vi "Original GenerateTestAllTask.vi"() -> (3 "Task Out":refnum<k21>)   [LabVIEW 2013]
uses:
  <vilib>/DAQmx/create/channels.llb/DAQmx Create Channel (AI-Voltage-Basic).vi
  <vilib>/DAQmx/create/channels.llb/DAQmx Create Channel (AI-Strain-Strain Gage).vi
  <vilib>/DAQmx/create/channels.llb/DAQmx Create Channel (AI-Position-LVDT).vi
  <vilib>/DAQmx/create/channels.llb/DAQmx Create Channel (AI-Position-RVDT).vi
  Instance           1 27Saved   GenerateTestAllTask .vi
  <resource>/objmgr/daqmx.rc
  Popups/Progress Bar Actions.ctl
panel:
  in  "Channel Path List":string[](array[string])
  out "error out":errorcluster
  in  "error in (no error)":errorcluster
  out "Name":string
  out "AI.MeasType":i32(ring)=10300 items=["Voltage"=10322, "Current"=10134, "More:Voltage:Custom with Excitation"=10323, "Frequency"=10181, "Resistance"=10278, "Temperature:Thermocouple"=10303, "Temperature:Thermistor"=10302, "Temperature:RTD"=10301, "Temperature:Built-in Sensor"=10311, "Strain Gage"=10300, "Position:LVDT"=10352, "Position:RVDT"=10353, "Accelerometer"=10356, "Sound Pressure:Microphone"=10354, "TEDS Sensor"=12531]
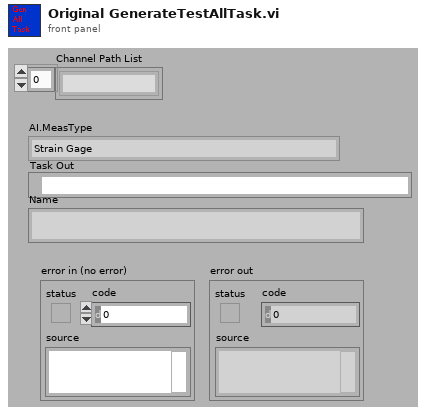
[diagram p1: front panel]
types:
  T1 = typedef "Progress Bar Actions.ctl" = enum16{"Get", "Set", "Exit", "Init"}
  T2 = cluster{"gage factor":dbl, "nominal gage resistance":dbl, "poisson ratio":dbl}
  T3 = cluster{"strain configuration":i32, "lead wire resistance":dbl, "initial bridge voltage":dbl, "voltage excitation source":i32, "voltage excitation value":dbl}
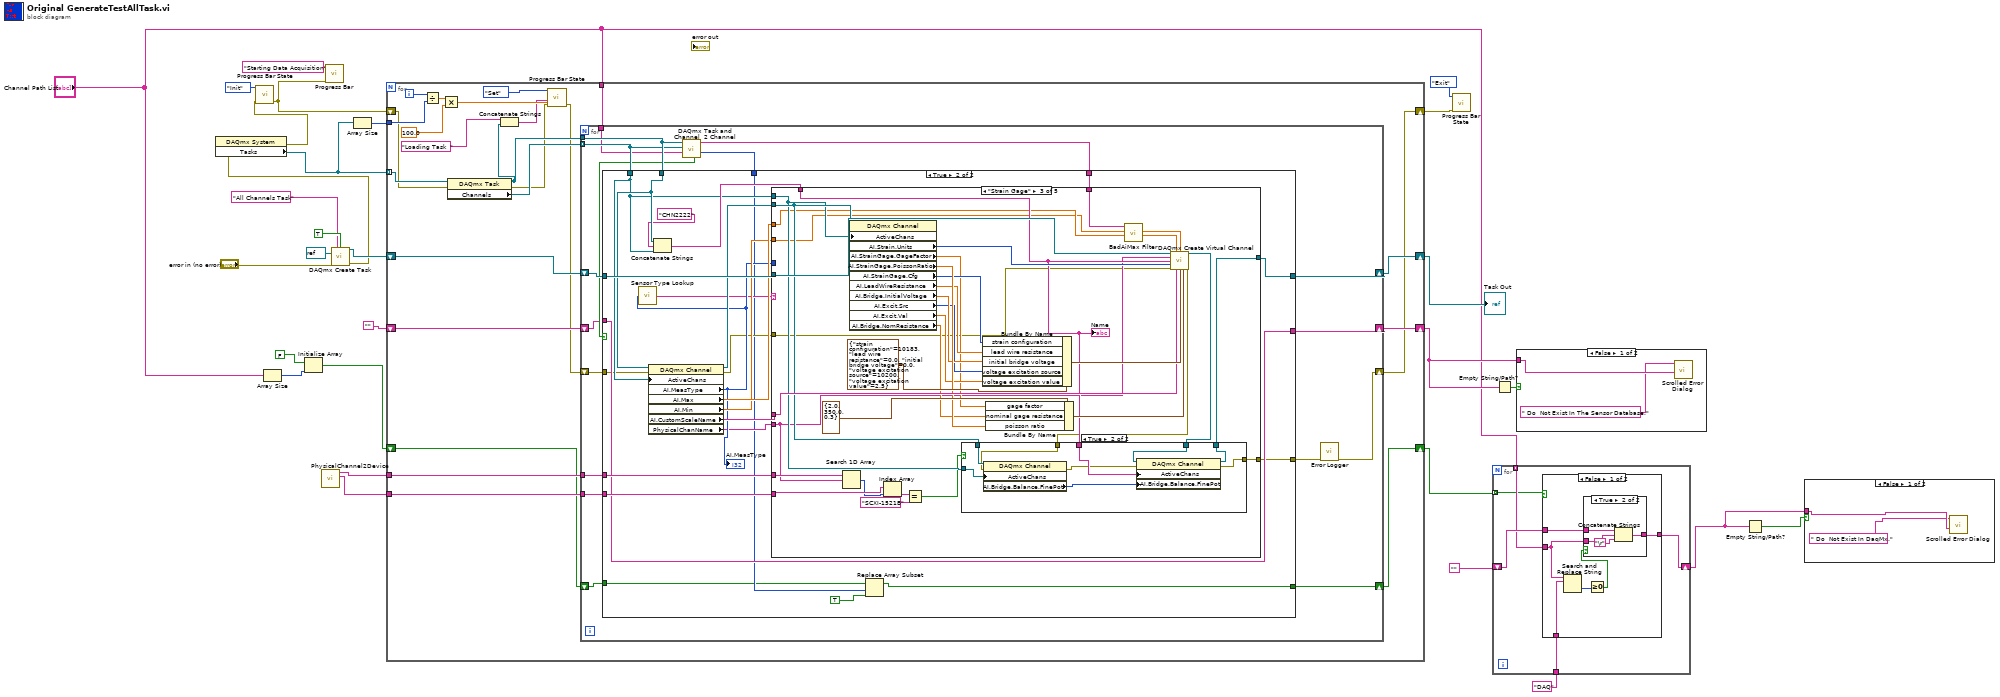
[diagram p0: block diagram]
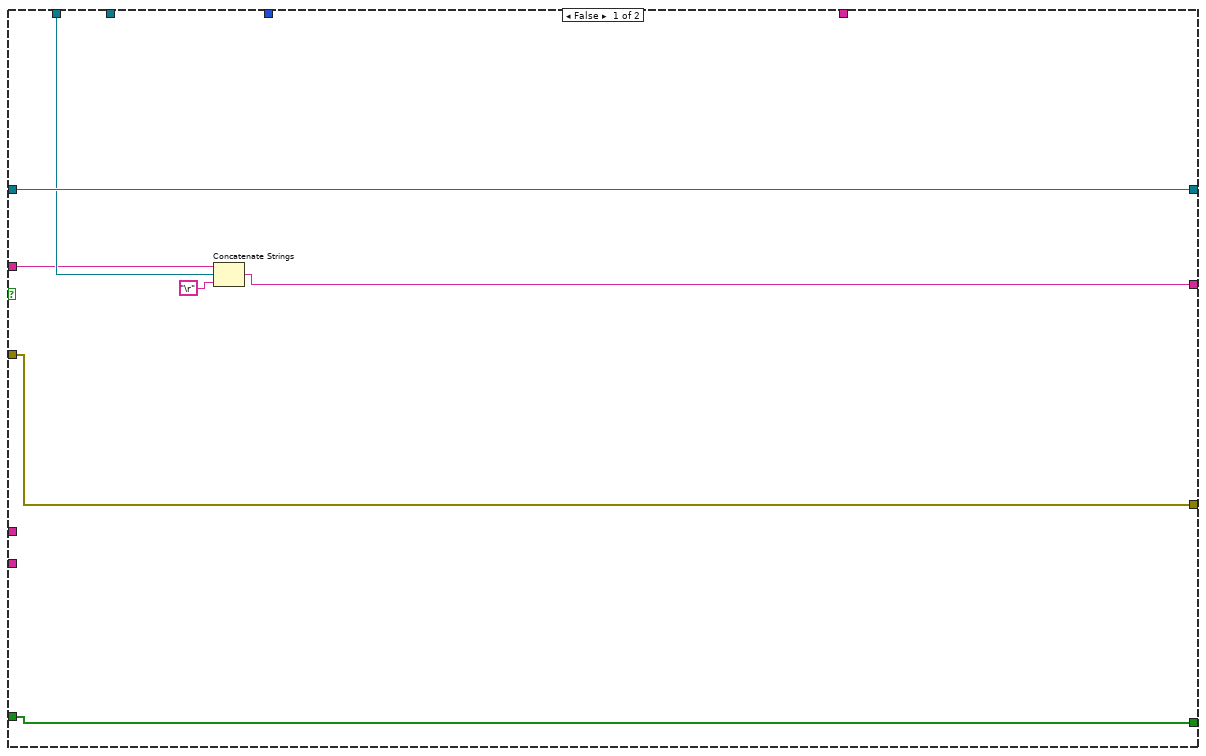
[diagram p6: hidden frame]
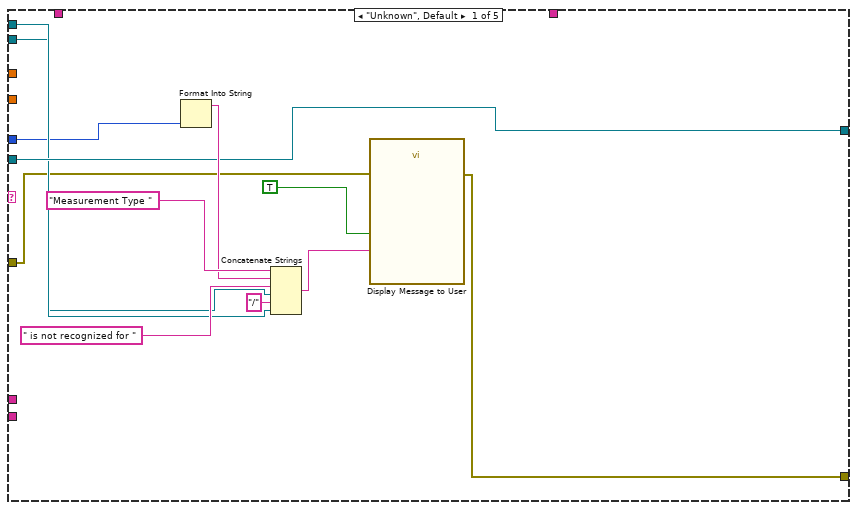
[diagram p7: hidden frame]
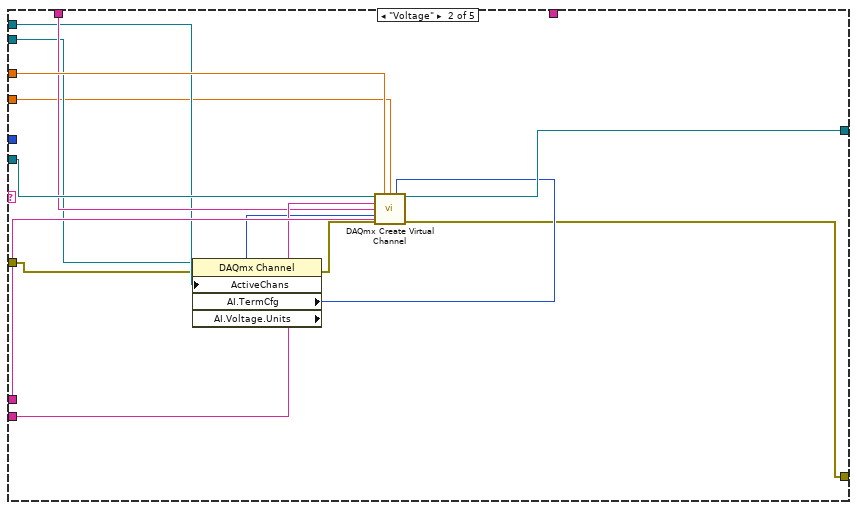
[diagram p8: hidden frame]
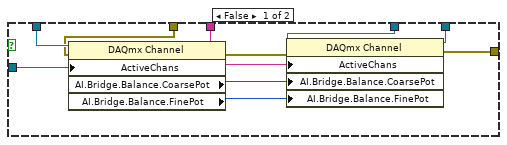
[diagram p9: hidden frame]
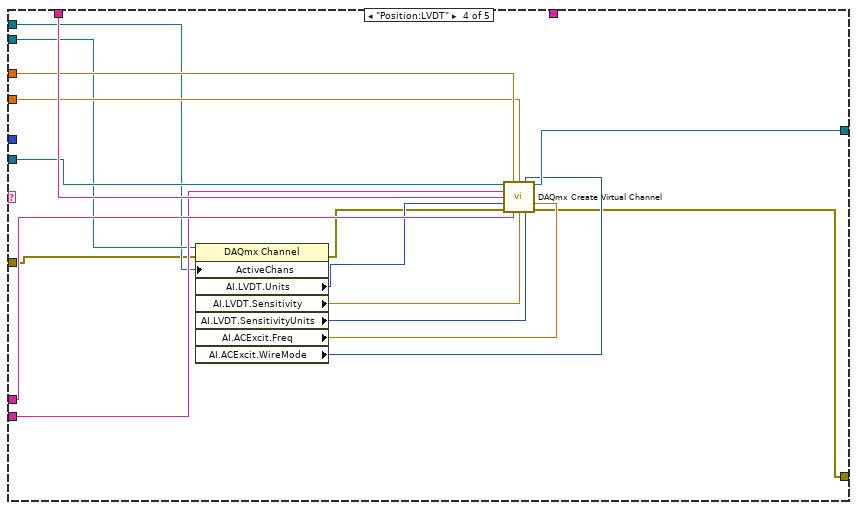
[diagram p10: hidden frame]
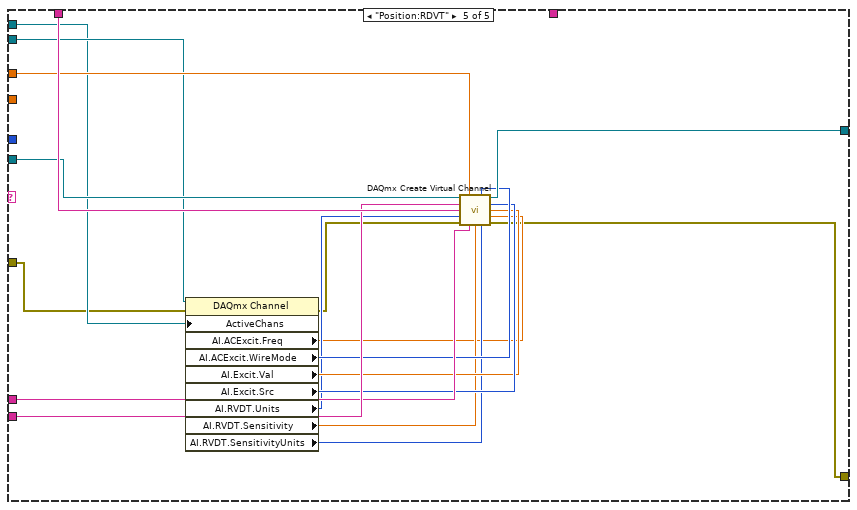
[diagram p11: hidden frame]
diagram:
  n1 = Array Size(array="Channel Path List") -> (size(s)=w10:i32)
  n2 = Initialize Array(FALSE, w10) -> (w8:bool[])
  n3 = call "PhysicalChannel2Device.vi"() -> ("Associated Device"=w23:string[], "Physical Channels"=w24:tag[])  [unwired: 10 out]
  n4 = call <vilib>:"DAQmx Create Task.vi"("new task name"="All Channels Task", "auto cleanup"=TRUE, "task to copy"=refnum<k21> refnum, "error in"="error in (no error)") -> ("task out"=w27:refnum<k21>, "error out"=w12:errorcluster)  [unwired: 1 in, 9 out]
  n5 = property class="DAQmx System"(error in=w12) -> (error out=w11:errorcluster, "Tasks"=w18:refnum<k21>[])  [unwired: 1 in, 1 out]
  n6 = call "Progress Bar State.vi"("error in (no error)"=w11, "Progress Actions"=Progress_Bar_Actions."Init") -> ("error out"=w14:errorcluster)  [unwired: 2 in, 7 out]
  n7 = call "Progress Bar.vi"("error in (no error)"=w14, "Label In"="Starting Data Acquisition") -> ()  [unwired: 10 out]
  n8 = Array Size(array=w18) -> (size(s)=w17:i32)
  n9 = for {
    tunnel: w18 -> [w53] mode=indexing
    shift-right: [w50] -> w26
    shift-left: w27 -> [w51]
    tunnel: w24 -> [w49]
    tunnel: w23 -> [w48]
    shift-right: [w46] -> w21
    shift-left: "" -> [w47]
    tunnel: w17 -> [w43]
    shift-right: [w32] -> w16
    shift-left: w14 -> [w35]
    tunnel: "Channel Path List" -> [w36]
    shift-right: [w30] -> w7
    shift-left: w8 -> [w31]
    i -> [w44]
    n10 = Divide(x=w44, y=w43) -> (x/y=w42:dbl)
    n11 = Multiply(x=w42, y=100.0) -> (x*y=w40:dbl)
    n12 = property class="DAQmx Task"(reference=w53, error in=w35) -> (reference out=w38:refnum<k21>, error out=w34:errorcluster, "Channels"=w52:refnum<k21>[])
    n13 = Concatenate Strings("Loading Task  " ("string"), w38) -> (w37:string)
    n14 = call "Progress Bar State.vi"("error in (no error)"=w34, "String In"=w37, "Progress In"=w40, "Progress Actions"=Progress_Bar_Actions."Set") -> ("error out"=w33:errorcluster)  [unwired: 7 out]
    n15 = for {
      tunnel: w52 -> [w67] mode=indexing
      tunnel: w38 -> [w68]
      shift-right: [w69] -> w50
      shift-left: w51 -> [w70]
      tunnel: w49 -> [w65]
      tunnel: w48 -> [w64]
      shift-right: [w62] -> w46
      shift-left: w47 -> [w63]
      tunnel: w36 -> [w61]
      shift-right: [w58] -> w32
      shift-left: w33 -> [w60]
      shift-right: [w54] -> w30
      shift-left: w31 -> [w55]
      n16 = call "DAQmx Task and Channel  2 Channel.vi"("Channel Path List In"=w61, "Channel In"=w67, "DAQmx Task Name"=w68) -> ("Channel Name Index"=w56:i32, "Channel Out"=w57:string, "Exists"=w66:bool)  [unwired: 6 out]
      n17 = case shown="True" w66 {
        tunnel: w70 -> [w77 w101]
        tunnel: [w77 w100] -> w69
        tunnel: w68 -> [_ w97]
        tunnel: w67 -> [w76 w94]
        tunnel: w65 -> [_ w88]
        tunnel: w64 -> [_ w87]
        tunnel: w63 -> [w74 w86]
        tunnel: [w73 w86] -> w62
        tunnel: w60 -> [w72 w85]
        tunnel: [w72 w83] -> w59
        tunnel: w57 -> [_ w82]
        tunnel: w56 -> [_ w81]
        tunnel: w55 -> [w71 w80]
        tunnel: [w71 w78] -> w54
        frame False {
          n18 = Concatenate Strings(w74, w76, "\r") -> (w73:string)
        }
        frame True {
          n19 = property class="DAQmx Channel"(reference=w97, error in=w85, "ActiveChans"=w94) -> (reference out=w93:refnum<k21>, error out=w84:errorcluster, "AI.MeasType"=w91:i32, "AI.Max"=w99:dbl, "AI.Min"=w92:dbl, "AI.CustomScaleName"=w98:tag, "PhysicalChanName"=w89:tag)
          "AI.MeasType" <- w91
          n20 = call "Sensor Type Lookup.vi"("AI.MeasType"=w91) -> ("String Rep"=w90:string)
          n21 = Concatenate Strings(w97, "CHN2222", w94) -> (w96:string)
          n22 = case shown="\"Strain Gage\"" w90 {
            tunnel: w101 -> [w108 w127 w162 w189 w214]
            tunnel: [w108 w126 w144 w194 w211] -> w100
            tunnel: w99 -> [_ w125 w129 w197 w215]
            tunnel: w98 -> [_ w124 w157 w196 w212]
            tunnel: w89 -> [_ w123 w140 w195 w213]
            tunnel: w96 -> [_ w122 w145 w198 w216]
            tunnel: w94 -> [w106 w121 w146 w185 w202]
            tunnel: w93 -> [w105 w118 w147 w187 w204]
            tunnel: w92 -> [_ w117 w128 w188 _]
            tunnel: w91 -> [w104 _ _ _ _]
            tunnel: w88 -> [_ _ w142 _ _]
            tunnel: w87 -> [_ _ w141 _ _]
            tunnel: w84 -> [w103 w116 w135 w184 w201]
            tunnel: [w102 w114 w133 w182 w199] -> w83
            tunnel: w82 -> [_ _ w132 _ _]
            frame "Unknown", Default {
              n23 = Format Into String(w104) -> (resulting string=w112:string)  [unwired: 3 in, 1 out]
              n24 = Concatenate Strings("Measurement Type " ("string"), w112, " is not recognized for " ("string"), w105, "/" ("string"), w106) -> (w110:string)
              n25 = call "Display Message to User"("error in (no error)"=w103, "Enable"=TRUE, "Message"=w110) -> ("error out"=w102:errorcluster)  [unwired: 8 out]
            }
            frame "Voltage" {
              n26 = property class="DAQmx Channel"(reference=w118, error in=w116, "ActiveChans"=w121) -> (error out=w115:errorcluster, "AI.TermCfg"=w120:i32, "AI.Voltage.Units"=w119:i32)  [unwired: 1 out]
              n27 = call-poly <vilib>:"DAQmx Create Virtual Channel.vi"("task in"=w127, "maximum value"=w125, "minimum value"=w117, "input terminal configuration"=w120, "physical channels"=w123, "name to assign"=w122, "units"=w119, "error in"=w115, "custom scale name"=w124) -> ("task out"=w126:refnum<k21>, "error out"=w114:errorcluster)  [unwired: 5 out]
            }
            frame "Strain Gage" {
              n28 = Search 1D Array(1D array=w142, element=w140) -> (index of element=w139:i32)  [unwired: 1 out]
              n29 = property class="DAQmx Channel"(reference=w147, "ActiveChans"=w146) -> ("AI.Strain.Units"=w150:i32, "AI.StrainGage.GageFactor"=w149:dbl, "AI.StrainGage.PoissonRatio"=w156:dbl, "AI.StrainGage.Cfg"=w155:i32, "AI.LeadWireResistance"=w154:dbl, "AI.Bridge.InitialVoltage"=w153:dbl, "AI.Excit.Src"=w152:i32, "AI.Excit.Val"=w151:dbl, "AI.Bridge.NomResistance"=w148:dbl)  [unwired: 1 in, 2 out]
              n30 = Index Array(array=w141, index=w139) -> (element=w138:string)
              n31 = Equal?(x=w138, y="SCXI-1521B") -> (x = y?=w136:bool)
              n32 = Bundle By Name(cluster=T3 {"strain configuration"=10183, "lead wire resistance"=0.0, "initial bridge voltage"=0.0, "voltage excitation source"=10200, "voltage excitation value"=2.5} ("bridge information"), "strain configuration"=w155, "lead wire resistance"=w154, "initial bridge voltage"=w153, "voltage excitation source"=w152, "voltage excitation value"=w151) -> (w160:T3)
              n33 = Bundle By Name(cluster=T2 {"gage factor"=2.0, "nominal gage resistance"=350.0, "poisson ratio"=0.3} ("strain gage information"), "gage factor"=w149, "nominal gage resistance"=w148, "poisson ratio"=w156) -> (w158:T2)
              n34 = call "BadAiMax Filter.vi"("Max In"=w129, "Min In"=w128, "Channel Name"=w132) -> ("Max Out"=w130:dbl, "Min Out"=w131:dbl)  [unwired: 6 in, 1 out]
              n35 = call-poly <vilib>:"DAQmx Create Virtual Channel.vi"("task in"=w162, "maximum value"=w130, "minimum value"=w131, "physical channels"=w140, "name to assign"=w145, "units"=w150, "error in"=w135, "custom scale name"=w157, "bridge information"=w160, "strain gage information"=w158) -> ("task out"=w143:refnum<k21>, "error out"=w134:errorcluster)  [unwired: 1 in, 3 out]
              n36 = case shown="True" w136 {
                tunnel: w147 -> [w172 w176]
                tunnel: w146 -> [w171 w177]
                tunnel: w145 -> [w170 w180]
                tunnel: w143 -> [w168 w179]
                tunnel: [w167 w178] -> w144
                tunnel: w134 -> [w165 w175]
                tunnel: [w163 w173] -> w133
                frame False {
                  n37 = property class="DAQmx Channel"(reference=w172, error in=w165, "ActiveChans"=w171) -> (error out=w164:errorcluster, "AI.Bridge.Balance.CoarsePot"=w169:i32, "AI.Bridge.Balance.FinePot"=w166:i32)  [unwired: 1 out]
                  n38 = property class="DAQmx Channel"(reference=w168, error in=w164, "ActiveChans"=w170, "AI.Bridge.Balance.CoarsePot"=w169, "AI.Bridge.Balance.FinePot"=w166) -> (reference out=w167:refnum<k21>, error out=w163:errorcluster)
                }
                frame True {
                  n39 = property class="DAQmx Channel"(reference=w176, error in=w175, "ActiveChans"=w177) -> (error out=w174:errorcluster, "AI.Bridge.Balance.FinePot"=w181:i32)  [unwired: 1 out]
                  n40 = property class="DAQmx Channel"(reference=w179, error in=w174, "ActiveChans"=w180, "AI.Bridge.Balance.FinePot"=w181) -> (reference out=w178:refnum<k21>, error out=w173:errorcluster)
                }
              }
              "Name" <- w145
            }
            frame "Position:LVDT" {
              n41 = property class="DAQmx Channel"(reference=w187, error in=w184, "ActiveChans"=w185) -> (error out=w183:errorcluster, "AI.LVDT.Units"=w186:i32, "AI.LVDT.Sensitivity"=w193:dbl, "AI.LVDT.SensitivityUnits"=w192:i32, "AI.ACExcit.Freq"=w191:dbl, "AI.ACExcit.WireMode"=w190:i32)  [unwired: 1 out]
              n42 = call-poly <vilib>:"DAQmx Create Virtual Channel.vi"("task in"=w189, "maximum value"=w197, "minimum value"=w188, "voltage excitation wire mode"=w190, "physical channels"=w195, "name to assign"=w198, "units"=w186, "voltage excitation frequency"=w191, "error in"=w183, "custom scale name"=w196, "sensitivity"=w193, "sensitivity units"=w192) -> ("task out"=w194:refnum<k21>, "error out"=w182:errorcluster)  [unwired: 2 in]
            }
            frame "Position:RDVT" {
              n43 = property class="DAQmx Channel"(reference=w204, error in=w201, "ActiveChans"=w202) -> (error out=w200:errorcluster, "AI.ACExcit.Freq"=w203:dbl, "AI.ACExcit.WireMode"=w210:i32, "AI.Excit.Val"=w208:dbl, "AI.Excit.Src"=w209:i32, "AI.RVDT.Units"=w207:i32, "AI.RVDT.Sensitivity"=w206:dbl, "AI.RVDT.SensitivityUnits"=w205:i32)  [unwired: 1 out]
              n44 = call-poly <vilib>:"DAQmx Create Virtual Channel.vi"("task in"=w214, "maximum value"=w215, "voltage excitation wire mode"=w210, "physical channels"=w213, "voltage excitation source"=w209, "name to assign"=w216, "voltage excitation value"=w208, "units"=w207, "voltage excitation frequency"=w203, "error in"=w200, "custom scale name"=w212, "sensitivity"=w206, "sensitivity units"=w205) -> ("task out"=w211:refnum<k21>, "error out"=w199:errorcluster)  [unwired: 1 in]
            }
          }
          n45 = Replace Array Subset(array=w80, new element=TRUE ("new element/subarray"), index=w81) -> (w78:bool[])
        }
      }
      n46 = call "Error Logger.vi"("error in (no error)"=w59) -> ("error out"=w58:errorcluster)  [unwired: 10 in]
    }
  }
  "Task Out" <- w26
  n47 = call "Progress Bar State.vi"("error in (no error)"=w16, "Progress Actions"=Progress_Bar_Actions."Exit") -> ()  [unwired: 2 in, 8 out]
  n48 = for {
    tunnel: "Channel Path List" -> [w219] mode=indexing
    tunnel: w7 -> [w218] mode=indexing
    shift-right: [w220] -> w4
    shift-left: "" -> [w221]
    tunnel: "DAQ" ("search string") -> [w217]
    n49 = case shown="False" w218 {
      tunnel: w219 -> [w225 _]
      tunnel: w221 -> [w227 w233]
      tunnel: [w226 w233] -> w220
      tunnel: w217 -> [w224 _]
      frame False {
        n50 = Search and Replace String(input string=w225, search string=w224) -> (offset past replacement=w223:i32)  [unwired: 6 in, 3 out]
        n51 = Greater Or Equal To 0?(x=w223) -> (x >= 0?=w222:bool)
        n52 = case shown="True" w222 {
          tunnel: w227 -> [w228 w231]
          tunnel: [w228 w230] -> w226
          tunnel: w225 -> [_ w229]
          frame False {
          }
          frame True {
            n53 = Concatenate Strings(w231, w229, "\r") -> (w230:string)
          }
        }
      }
      frame True {
      }
    }
  }
  n54 = Empty String/Path?(string/path=w21) -> (empty?=w22:bool)
  n55 = case shown="False" w22 {
    tunnel: w21 -> [w235 _]
    frame False {
      n56 = call "Scrolled Error Dialog.vi"("Channels"=w235, "Title"=" Do  Not Exist In The Sensor Database." ("string")) -> ()  [unwired: 9 in, 1 out]
    }
    frame True {
    }
  }
  n57 = Empty String/Path?(string/path=w4) -> (empty?=w5:bool)
  n58 = case shown="False" w5 {
    tunnel: w4 -> [w237 _]
    frame False {
      n59 = call "Scrolled Error Dialog.vi"("Channels"=w237, "Title"=" Do  Not Exist In DaqMx." ("string")) -> ()  [unwired: 9 in, 1 out]
    }
    frame True {
    }
  }
